vi "Pfeiffer_DPG_202_Pressure_Readout_Once.vi"(11 "VISA session in":refnum<visa-resource-name>) -> (0 "Pressure Ch 2":dbl format="%_3e", 1 "Pressure Ch 1":dbl format="%_3e", 2 "Pressure Ch 2":string, 3 "Pressure Ch 1":string)   [LabVIEW 2013]
uses:
  Pfeiffer Vacuum/Public/DigiLine/Digiline - Cluster.ctl
  Pfeiffer Vacuum/Pfeiffer Vacuum.lvlib
panel:
  out "error out":errorcluster
  in  "error in (no error)":errorcluster
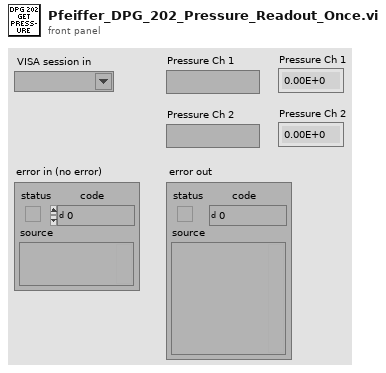
[diagram p1: front panel]
types:
  T1 = typedef "Pfeiffer Vacuum.lvlib/Digiline - Cluster.ctl" = cluster{"Parameter":u16, "Parameter\nread only<->describe":bool, "Correction facktor\n(0,20 - 9,90) ":sgl, "Pressure set point (mbar)\n0 ==> ur (p<1,0e-4 mbar)\n1 - 2050 mbar":i16}
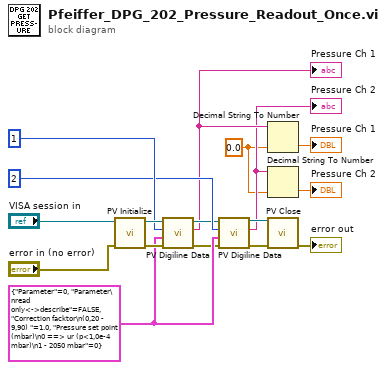
[diagram p0: block diagram]
diagram:
  w3 = 0.0 ("default (0 I32)")
  w9 = T1 {"Parameter"=0, "Parameter\nread only<->describe"=FALSE, "Correction facktor\n(0,20 - 9,90) "=1.0, "Pressure set point (mbar)\n0 ==> ur (p<1,0e-4 mbar)\n1 - 2050 mbar"=0} ("DigiLine-Cluster")
  n1 = call "PV Initialize.vi"("error in (no error)"="error in (no error)", "VISA session in"="VISA session in") -> ("error out"=w17:errorcluster, "VISA session out"=w16:refnum<visa-resource-name>)  [unwired: 8 in]
  n2 = call "PV Digiline Data.vi"("error in (no error)"=w17, "DigiLine-Cluster"=w9, "Adress of unit"=u16 1 ("Ch 1"), "VISA session"=w16) -> ("error out"=w6:errorcluster, "response (data)"=w5:string, "dup VISA session"=w7:refnum<visa-resource-name>)  [unwired: 5 in]
  "Pressure Ch 1" <- w5
  n3 = call "PV Digiline Data.vi"("error in (no error)"=w6, "DigiLine-Cluster"=w9, "Adress of unit"=u16 2 ("Ch 2"), "VISA session"=w7) -> ("error out"=w11:errorcluster, "response (data)"=w4:string, "dup VISA session"=w12:refnum<visa-resource-name>)  [unwired: 5 in]
  "Pressure Ch 2" <- w4
  n4 = Decimal String To Number(string=w5, default (0L)=w3) -> (number=→"Pressure Ch 1":dbl)  [unwired: 1 in, 1 out]
  n5 = Decimal String To Number(string=w4, default (0L)=w3) -> (number=→"Pressure Ch 2":dbl)  [unwired: 1 in, 1 out]
  n6 = call "PV Close.vi"("VISA session"=w12, "error in (no error)"=w11) -> ("error out"=→"error out":errorcluster)  [unwired: 13 in]
